vi "Calculate average rate.vi"(8 "error in (no error)":errorcluster, 11 "Automatic Mode in":refnum<class "Automatic Mode.lvclass">) -> (0 "error out":errorcluster, 2 "Average rate":dbl, 3 "Automatic Mode out":refnum<class "Automatic Mode.lvclass">)   [LabVIEW 2015, in "Automatic Mode.lvclass"]
uses:
  Automatic Mode.lvclass
  Automatic Mode.lvclass/Automatic Mode.ctl
  <vilib>/Analysis/baseanly.llb/Mean (DBL).vi
  <vilib>/Analysis/NI_AALBase.lvlib
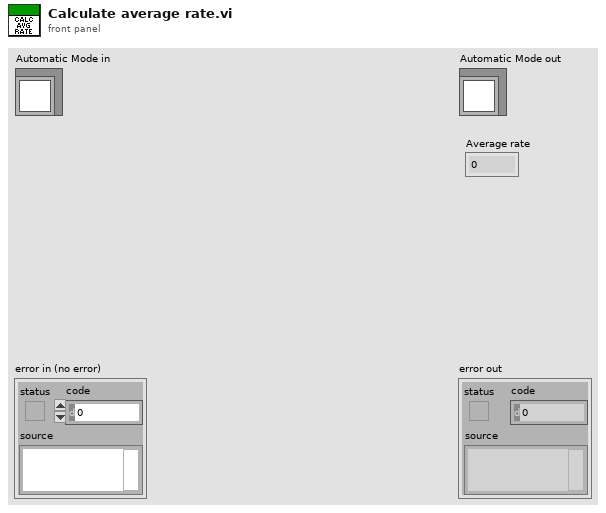
[diagram p1: front panel]
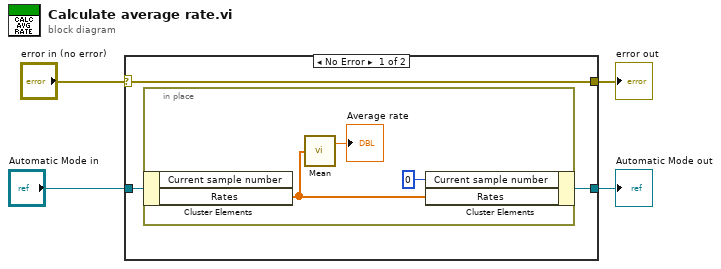
[diagram p0: block diagram]
diagram:
  n1 = case shown="No Error" "error in (no error)" {
    selector: "error in (no error)" -> [w7 w12]
    tunnel: [w7 w12] -> w3
    tunnel: [w5 w11] -> w1
    tunnel: "Automatic Mode in" -> [w6 w11]
    frame No Error {
      n2 = in-place {
        n3 = in-place-cluster #1(w6) -> ("Rates"=w8:dbl[])  [unwired: 1 out]
        n4 = call-poly <vilib>:"Mean.vi"("X"=w8) -> ("mean"=→"Average rate":dbl)  [unwired: 1 out]
        n5 = in-place-cluster #1("Current sample number"=0, "Rates"=w8) -> (w5:refnum<class "Automatic Mode.lvclass">)
      }
    }
    frame Error {
    }
  }
  "error out" <- w3
  "Automatic Mode out" <- w1
